vi "Teleop Drivetrain Control.vi"(9 "Driver D-Pad Cluster":T1, 10 "Driver Button Cluster":T2, 11 "Driver Axes Cluster":T3) -> ()   [LabVIEW 2016]
uses:
  Common Code/Gamepads/Axes Cluster.ctl
  Common Code/Gamepads/Button Cluster.ctl
  Common Code/Gamepads/D-Pad.ctl
  Common Code/Utilities/Change Detect.vi
  Common Code/Utilities/Change Detect Boolean.vi
  Robot Global Data.vi
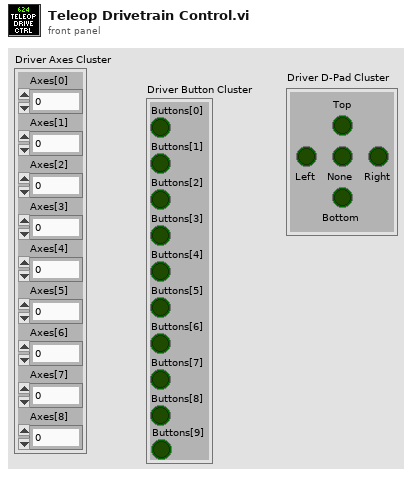
[diagram p1: front panel]
types:
  T1 = typedef "D-Pad.ctl" = cluster{"Top":bool, "Bottom":bool, "None":bool, "Right":bool, "Left":bool}
  T2 = typedef "Button Cluster.ctl" = cluster{"Buttons[0]":bool, "Buttons[1]":bool, "Buttons[2]":bool, "Buttons[3]":bool, "Buttons[4]":bool, "Buttons[5]":bool, "Buttons[6]":bool, "Buttons[7]":bool, "Buttons[8]":bool, "Buttons[9]":bool}
  T3 = typedef "Axes Cluster.ctl" = cluster{"Axes[0]":dbl, "Axes[1]":dbl, "Axes[2]":dbl, "Axes[3]":dbl, "Axes[4]":dbl, "Axes[5]":dbl, "Axes[6]":dbl, "Axes[7]":dbl, "Axes[8]":dbl}
  T4 = typedef "Dashboard Control Data.ctl" = cluster{"Drivetrain Settings":T5, "Intake Presets ":T7, "Drivetrain Encoder Settings":T8}
  T5 = typedef "Drivetrain Settings.ctl" = cluster{"Gyro Tolerance":dbl, "Gyro Steer PID Gains":T6, "Y Power Multiplier":dbl, "Turn Power Multiplier":dbl, "Gyro Output":dbl, "Creep Rate":dbl, "Distance Drive PID Gains":T6, "Distance Tolerance":dbl, "Distance Output":dbl, "Strafe Threshold":dbl, "Strafe Correct":bool, "Strafe Corect Tolerance":dbl, "Translate Drive PID Gains":T6, "Strafe Output":dbl}
  T6 = typedef "PID Gains.ctl" = cluster{"proportional gain (Kc)":dbl, "integral time (Ti, min)":dbl, "derivative time (Td, min)":dbl}
  T7 = typedef "Intake Presets.ctl" = cluster{"Intake Speed ":dbl, "Outake Speed":dbl, "Set Time":dbl}
  T8 = typedef "Drivetrain Encoder Settings.ctl" = cluster{"Left Tick Constant":dbl, "Right Tick Contant":dbl, "Reset Encoders":bool, "Center Tick Constant":dbl}
  T9 = typedef "Drivetrain Command Cluster.ctl" = cluster{"Drivetrain Mode":T10, "Heading Target":dbl, "Turn Power":dbl, "Y Power":dbl, "Center Piston Down?":bool, "Traction?":bool, "Strafe Power":dbl, "Zero Gyro":bool, "Distance Target":dbl, "Strafe Correct":bool, "Y Max Output":dbl, "Y Min Output":dbl, "X Max Output":dbl, "X Min Output":dbl, "Z Max Output":dbl, "Z Min Output":dbl, "Z Target":dbl}
  T10 = typedef "Drivetrain Mode.ctl" = enum16{"Manual", "Gyro Steer", "Distance Drive", "Translate Drive", "PID Drive"}
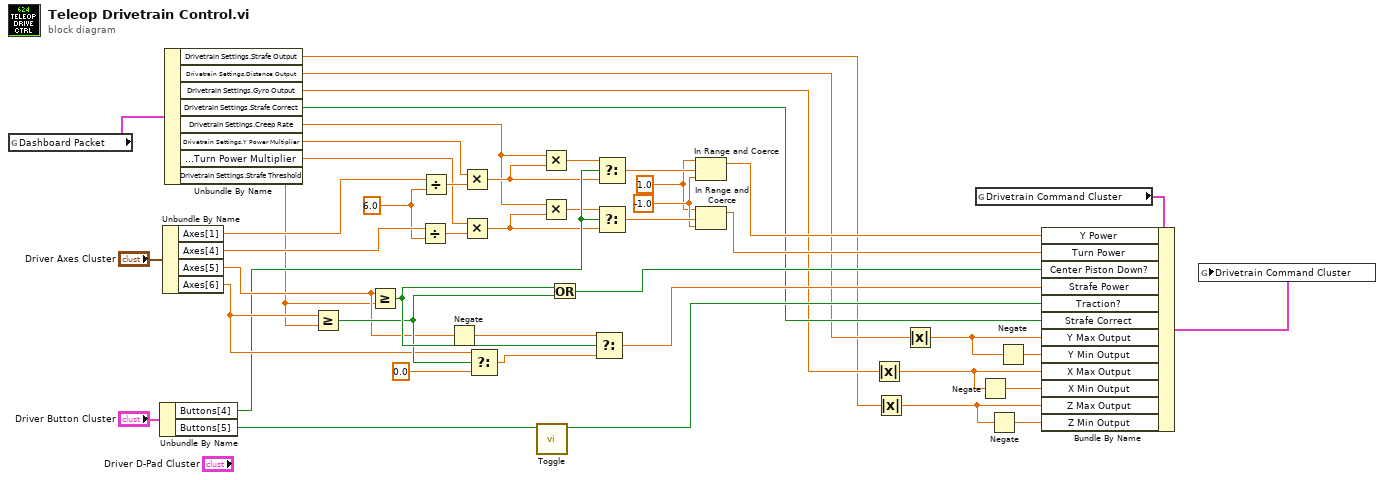
[diagram p0: block diagram]
diagram:
  w13 = 1.0 ("upper limit")
  w15 = -1.0 ("lower limit")
  w27 = 6.0 ("y")
  n1 = global read "Robot Global Data.vi" "Dashboard Packet"() -> (w14:T4)
  n2 = Unbundle By Name("Driver Button Cluster") -> ("Buttons[4]"=w34:bool, "Buttons[5]"=w33:bool)
  n3 = Unbundle By Name("Driver Axes Cluster") -> ("Axes[1]"=w36:dbl, "Axes[4]"=w35:dbl, "Axes[5]"=w40:dbl, "Axes[6]"=w38:dbl)
  n4 = Unbundle By Name(w14) -> ("Drivetrain Settings.Strafe Output"=w3:dbl, "Drivetrain Settings.Distance Output"=w9:dbl, "Drivetrain Settings.Gyro Output"=w8:dbl, "Drivetrain Settings.Strafe Correct"=w10:bool, "Drivetrain Settings.Creep Rate"=w12:dbl, "Drivetrain Settings.Y Power Multiplier"=w26:dbl, "Drivetrain Settings.Turn Power Multiplier"=w25:dbl, "Drivetrain Settings.Strafe Threshold"=w11:dbl)
  n5 = Greater Or Equal?(x=w38, y=w11) -> (x >= y?=w42:bool)
  n6 = Greater Or Equal?(x=w40, y=w11) -> (x >= y?=w45:bool)
  n7 = Divide(x=w35, y=w27) -> (x/y=w28:dbl)
  n8 = Divide(x=w36, y=w27) -> (x/y=w29:dbl)
  n9 = Negate(x=w40) -> (-x=w39:dbl)
  n10 = Multiply(x=w26, y=w29) -> (x*y=w24:dbl)
  n11 = Multiply(x=w25, y=w28) -> (x*y=w20:dbl)
  n12 = Select(t=w38, s=w42, f=0.0) -> (s? t:f=w43:dbl)
  n13 = call "Toggle.vi"("In"=w33) -> ("Toggled"=w30:bool)  [unwired: 10 in]
  n14 = Multiply(x=w12, y=w24) -> (x*y=w23:dbl)
  n15 = Multiply(x=w12, y=w20) -> (x*y=w21:dbl)
  n16 = Or(x=w45, y=w42) -> (x .or. y?=w44:bool)
  n17 = Select(t=w39, s=w45, f=w43) -> (s? t:f=w41:dbl)
  n18 = Select(t=w23, s=w34, f=w24) -> (s? t:f=w31:dbl)
  n19 = Select(t=w21, s=w34, f=w20) -> (s? t:f=w16:dbl)
  n20 = In Range and Coerce(upper limit=w13, x=w31, lower limit=w15) -> (coerced(x)=w18:dbl)  [unwired: 1 out]
  n21 = In Range and Coerce(upper limit=w13, x=w16, lower limit=w15) -> (coerced(x)=w17:dbl)  [unwired: 1 out]
  n22 = Absolute Value(x=w8) -> (abs(x)=w7:dbl)
  n23 = Absolute Value(x=w3) -> (abs(x)=w2:dbl)
  n24 = Absolute Value(x=w9) -> (abs(x)=w6:dbl)
  n25 = global read "Robot Global Data.vi" "Drivetrain Command Cluster"() -> (w22:T9)
  n26 = Negate(x=w7) -> (-x=w5:dbl)
  n27 = Negate(x=w2) -> (-x=w1:dbl)
  n28 = Negate(x=w6) -> (-x=w4:dbl)
  n29 = Bundle By Name(cluster=w22, "Y Power"=w18, "Turn Power"=w17, "Center Piston Down?"=w44, "Strafe Power"=w41, "Traction?"=w30, "Strafe Correct"=w10, "Y Max Output"=w6, "Y Min Output"=w4, "X Max Output"=w7, "X Min Output"=w5, "Z Max Output"=w2, "Z Min Output"=w1) -> (w19:T9)
  n30 = global write "Robot Global Data.vi" "Drivetrain Command Cluster"(w19) -> ()
